vi "parse property names into string text.vi"(0 "String in":string, 4 "Property names":string, 5 "error in (no error)":errorcluster, 9 "Counter":i32) -> (14 "String out":string, 19 "error out":errorcluster)   [LabVIEW 2019, in "metadata.lvclass"]
doc: "parses the property names into a string text to view the property names and parameters side by side"
uses:
  metadata.lvclass
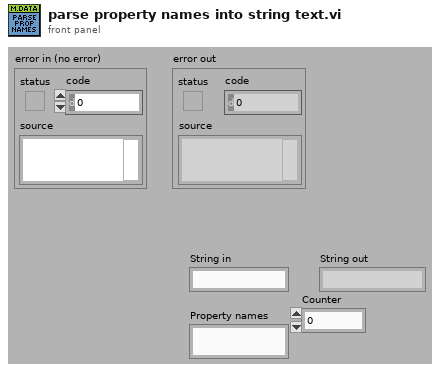
[diagram p1: front panel]
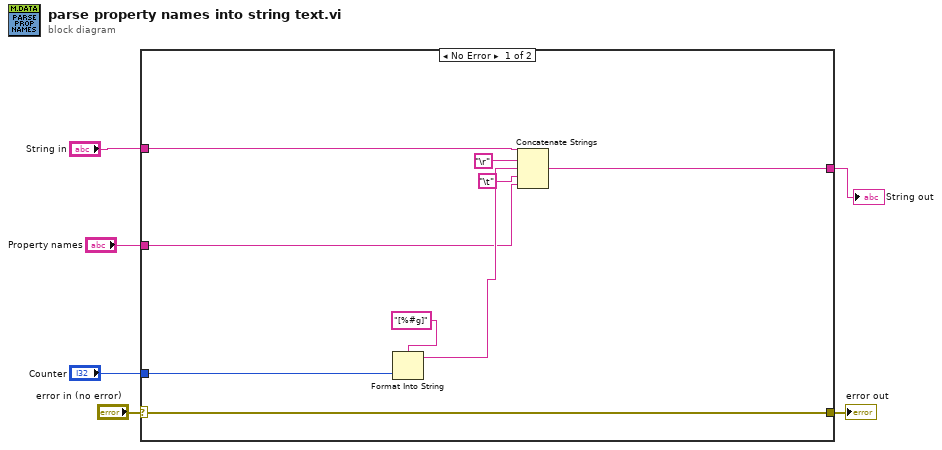
[diagram p0: block diagram]
diagram:
  n1 = case shown="No Error" "error in (no error)" {
    selector: "error in (no error)" -> [w15 w17]
    tunnel: [w15 w17] -> w5
    tunnel: [w10 w16] -> w4
    tunnel: "String in" -> [w9 w16]
    tunnel: "Counter" -> [w8 _]
    tunnel: "Property names" -> [w7 _]
    frame No Error {
      n2 = Format Into String(format string="[%#g]", w8) -> (resulting string=w13:string)  [unwired: 2 in, 1 out]
      n3 = Concatenate Strings(w9, "\r", w13, "\t", w7) -> (w10:string)
    }
    frame Error {
    }
  }
  "error out" <- w5
  "String out" <- w4
